vi "GetMethodExplicitName.vi"(8 "error in (no error)":errorcluster, 9 "options":i32 format="%.0x", 10 "method":string, 11 "Driver in":refnum<class "ViPER.lvclass">) -> (0 "error out":errorcluster, 1 "class explicit name":string, 2 "method explicit name":string, 3 "Driver out":refnum<class "ViPER.lvclass">, 4 "class":string, 5 "exists":bool, 6 "vi reference":refnum<vi>)   [LabVIEW 2022 SP3, in "ViPER.lvlib" / "ViPER.lvclass"]
doc: "### BSD License (http://www.opensource.org/licenses/bsd-license.php) Begin ###\n\nCopyright (c) 2018 Kurt Friday www.medulla.net\n\nAll rights reserved.\n\nRedistribution and use in source and binary forms, with or without\nmodification, are permitted provided that the following conditions are met:\n\n * Redistributions of source code must retain the above copyright\n notice, this list of conditions and the following disclaimer.\n\n * Redistributions in binary form must reproduce the above copyright\n notice, this list of conditions and the following disclaimer in the\n documentation and/or other materials provided with the distribution.\n\n * Neither the name of the <organization> nor the\n names of its contributors may be used to endorse or promote products\n derived from this software without specific prior written permission.\n\nTHIS SOFTWARE IS PROVIDED BY THE COPYRIGHT HOLDERS AND CONTRIBUTORS \"AS IS\" AND\nANY EXPRESS OR IMPLIED WARRANTIES, INCLUDING, BUT NOT LIMITED TO, THE IMPLIED\nWARRANTIES OF MERCHANTABILITY AND FITNESS FOR A PARTICULAR PURPOSE ARE\nDISCLAIMED. IN NO EVENT SHALL <COPYRIGHT HOLDER> BE LIABLE FOR ANY\nDIRECT, INDIRECT, INCIDENTAL, SPECIAL, EXEMPLARY, OR CONSEQUENTIAL DAMAGES\n(INCLUDING, BUT NOT LIMITED TO, PROCUREMENT OF SUBSTITUTE GOODS OR SERVICES;\nLOSS OF USE, DATA, OR PROFITS; OR BUSINESS INTERRUPTION) HOWEVER CAUSED AND\nON ANY THEORY OF LIABILITY, WHETHER IN CONTRACT, STRICT LIABILITY, OR TORT\n(INCLUDING NEGLIGENCE OR OTHERWISE) ARISING IN ANY WAY OUT OF THE USE OF THIS\nSOFTWARE, EVEN IF ADVISED OF THE POSSIBILITY OF SUCH DAMAGE."
uses:
  ViPER.lvclass
panel:
  # "### BSD License (http://www.opensource.org/licenses/bsd-license.php) Begin ###\n\nCopyright (c) 2018  Kurt Friday www.medulla.net\n\nAll rights reserved.\n\nRedistribution and use in source and binary forms, with or without\nmodification, are permitted provided that the following conditions are met:\n\n    * Redistributions of source code must retain the above copyright\n      notice, this list of conditions and the following disclaimer.\n\n    * Redistributions in binary form must reproduce the above copyright\n      notice, this list of conditions and the following disclaimer in the\n      documentation and/or other materials provided with the distribution.\n\n    * Neither the name of the <organization> nor the\n      names of its contributors may be used to endorse or promote products\n      derived from this software without specific prior written permission.\n\nTHIS SOFTWARE IS PROVIDED BY THE COPYRIGHT HOLDERS AND CONTRIBUTORS \"AS IS\" AND\nANY EXPRESS OR IMPLIED WARRANTIES, INCLUDING, BUT NOT LIMITED TO, THE IMPLIED\nWARRANTIES OF MERCHANTABILITY AND FITNESS FOR A PARTICULAR PURPOSE ARE\nDISCLAIMED. IN NO EVENT SHALL <COPYRIGHT HOLDER> BE LIABLE FOR ANY\nDIRECT, INDIRECT, INCIDENTAL, SPECIAL, EXEMPLARY, OR CONSEQUENTIAL DAMAGES\n(INCLUDING, BUT NOT LIMITED TO, PROCUREMENT OF SUBSTITUTE GOODS OR SERVICES;\nLOSS OF USE, DATA, OR PROFITS; OR BUSINESS INTERRUPTION) HOWEVER CAUSED AND\nON ANY THEORY OF LIABILITY, WHETHER IN CONTRACT, STRICT LIABILITY, OR TORT\n(INCLUDING NEGLIGENCE OR OTHERWISE) ARISING IN ANY WAY OUT OF THE USE OF THIS\nSOFTWARE, EVEN IF ADVISED OF THE POSSIBILITY OF SUCH DAMAGE."
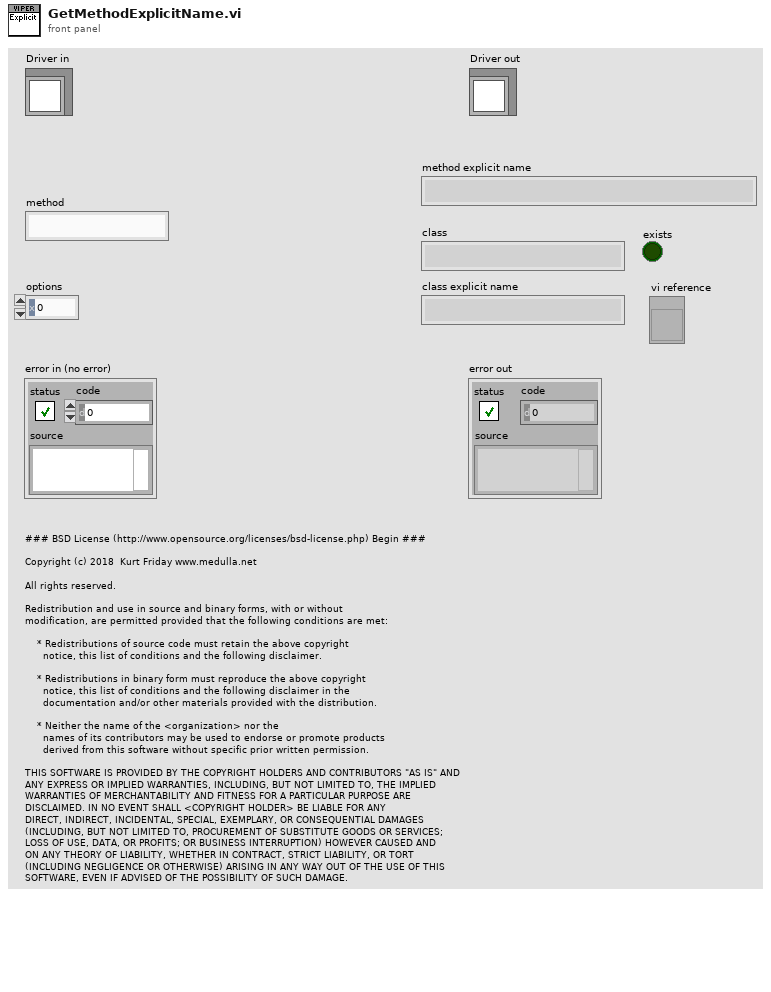
[diagram p1: front panel]
types:
  T1 = typedef "ViPER.lvlib/ViPER.lvclass/ObjectAttributes.ctl" = cluster{"Object":T2, "Ancestors":T4[], "Config":T5, "Init_OK":bool, "Hierachy":string[], "PPL?":bool[], "SFP_Open":bool[], "Config_SFP_Open":bool[], "SoftFP_event":refnum<user-event>[], "ConfigFP_event":refnum<user-event>[], "SoftFP_Shutdown_Notifier":refnum<notifier>[], "ConfigFP_Shutdown_Notifier":refnum<notifier>[]}
  T2 = typedef "ViPER.lvlib/ViPER.lvclass/ObjectDefinition.ctl" = cluster{"Name":string, "Ancestors":T3[]}
  T3 = typedef "ViPER.lvlib/ViPER.lvclass/Ancestor.ctl" = cluster{"Class":string, "Config":string, "Objects":string[]}
  T4 = typedef "ViPER.lvlib/ViPER.lvclass/ObjectLayers.ctl" = cluster{"Ancestor":string, "Objects":refnum<class "ViPER.lvclass">[], "Object_Names":string[], "Owned":bool[]}
  T5 = typedef "ViPER.lvlib/ViPER.lvclass/Config.ctl" = cluster{"default":string}
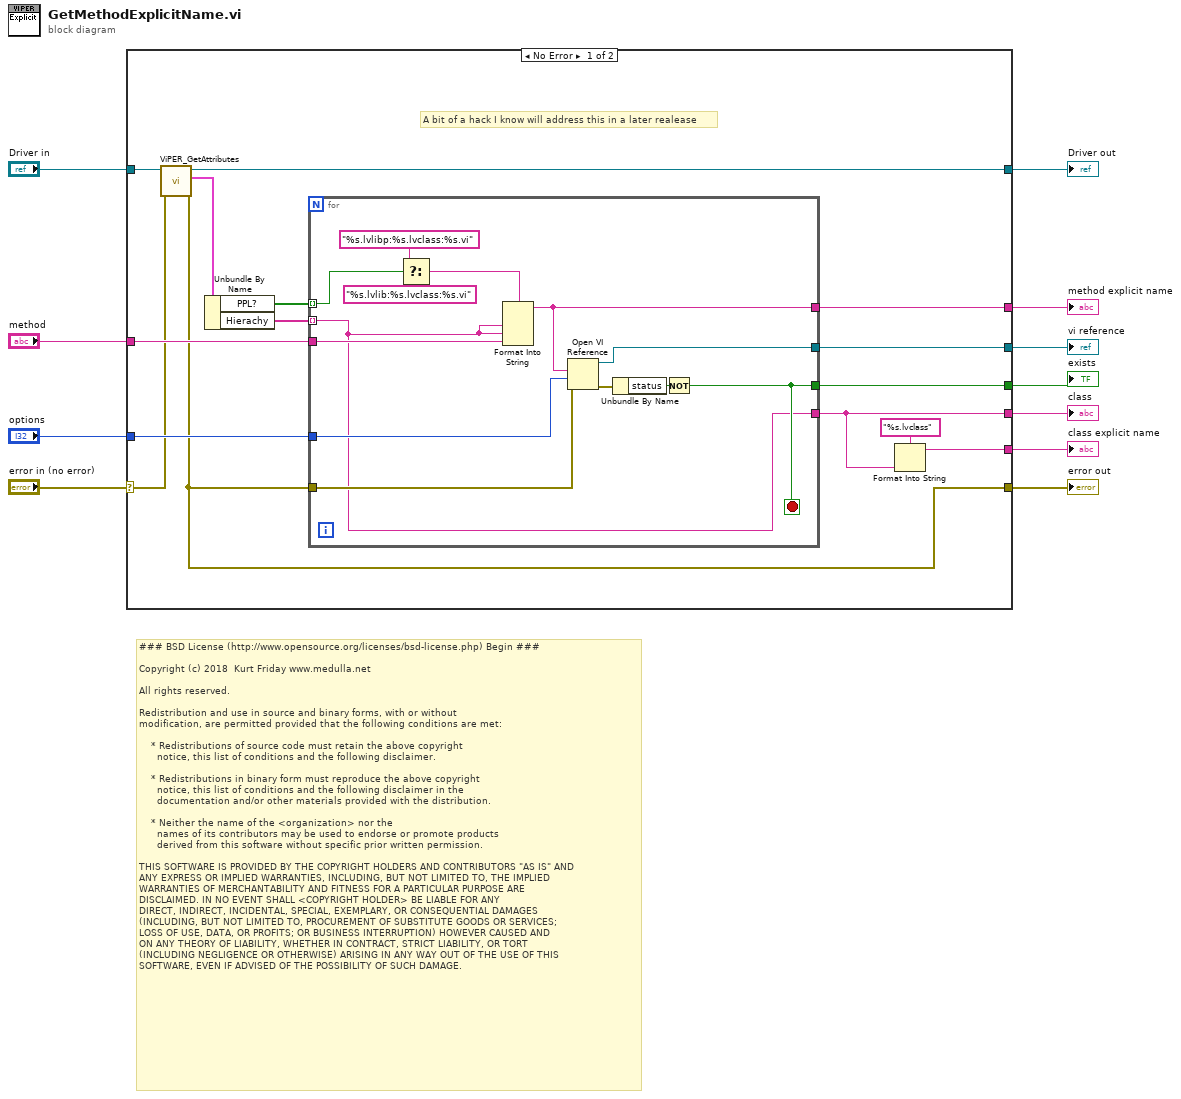
[diagram p0: block diagram]
diagram:
  # "### BSD License (http://www.opensource.org/licenses/bsd-license.php) Begin ###\n\nCopyright (c) 2018  Kurt Friday www.medulla.net\n\nAll rights reserved.\n\nRedistribution and use in source and binary forms, with or without\nmodification, are permitted provided that the following conditions are met:\n\n    * Redistributions of source code must retain the above copyright\n      notice, this list of conditions and the following disclaimer.\n\n    * Redistributions in binary form must reproduce the above copyright\n      notice, this list of conditions and the following disclaimer in the\n      documentation and/or other materials provided with the distribution.\n\n    * Neither the name of the <organization> nor the\n      names of its contributors may be used to endorse or promote products\n      derived from this software without specific prior written permission.\n\nTHIS SOFTWARE IS PROVIDED BY THE COPYRIGHT HOLDERS AND CONTRIBUTORS \"AS IS\" AND\nANY EXPRESS OR IMPLIED WARRANTIES, INCLUDING, BUT NOT LIMITED TO, THE IMPLIED\nWARRANTIES OF MERCHANTABILITY AND FITNESS FOR A PARTICULAR PURPOSE ARE\nDISCLAIMED. IN NO EVENT SHALL <COPYRIGHT HOLDER> BE LIABLE FOR ANY\nDIRECT, INDIRECT, INCIDENTAL, SPECIAL, EXEMPLARY, OR CONSEQUENTIAL DAMAGES\n(INCLUDING, BUT NOT LIMITED TO, PROCUREMENT OF SUBSTITUTE GOODS OR SERVICES;\nLOSS OF USE, DATA, OR PROFITS; OR BUSINESS INTERRUPTION) HOWEVER CAUSED AND\nON ANY THEORY OF LIABILITY, WHETHER IN CONTRACT, STRICT LIABILITY, OR TORT\n(INCLUDING NEGLIGENCE OR OTHERWISE) ARISING IN ANY WAY OUT OF THE USE OF THIS\nSOFTWARE, EVEN IF ADVISED OF THE POSSIBILITY OF SUCH DAMAGE."
  n1 = case shown="No Error" "error in (no error)" {
    selector: "error in (no error)" -> [w15 w41]
    tunnel: [w14 w41] -> w10
    tunnel: [w23 w40] -> w8
    tunnel: "Driver in" -> [w24 w40]
    tunnel: "method" -> [w21 _]
    tunnel: [w12 _] -> w6
    tunnel: [w16 _] -> w5
    tunnel: [w17 _] -> w4
    tunnel: [w26 _] -> w3
    tunnel: "options" -> [w25 _]
    tunnel: [w19 _] -> w1
    frame No Error {
      # "A bit of a hack I know will address this in a later realease"
      n2 = call "ViPER_GetAttributes.vi"("error in (no error)"=w15, "reference in"=w24) -> ("error out"=w14:errorcluster, "Data"=w22:T1, "reference out"=w23:refnum<class "ViPER.lvclass">)  [unwired: 6 in, 1 out]
      n3 = Unbundle By Name(w22) -> ("PPL?"=w13:bool[], "Hierachy"=w18:string[])
      n4 = for {
        tunnel: [w34] -> w16
        tunnel: [w39] -> w26
        tunnel: w25 -> [w38]
        tunnel: [w35] -> w17
        tunnel: w18 -> [w34] mode=indexing
        tunnel: w21 -> [w37]
        tunnel: w14 -> [w36]
        tunnel: [w27] -> w12
        tunnel: w13 -> [w33] mode=indexing
        stop <- w35 stop-if-true
        n5 = Select(t="%s.lvlibp:%s.lvclass:%s.vi", s=w33, f="%s.lvlib:%s.lvclass:%s.vi") -> (s? t:f=w28:string)
        n6 = Format Into String(format string=w28, w34, w34, w37) -> (resulting string=w27:string)  [unwired: 2 in, 1 out]
        n7 = Open VI Reference(vi path=w27, options=w38, error in (no error)=w36) -> (vi reference=w39:refnum<vi>, error out=w32:errorcluster)  [unwired: 3 in]
        n8 = Unbundle By Name(w32) -> ("status"=w31:bool)
        n9 = Not(x=w31) -> (.not. x?=w35:bool)
      }
      n10 = Format Into String(format string="%s.lvclass" ("regular expression"), w16) -> (resulting string=w19:string)  [unwired: 2 in, 1 out]
    }
    frame Error {
    }
  }
  "error out" <- w10
  "Driver out" <- w8
  "method explicit name" <- w6
  "class" <- w5
  "class explicit name" <- w1
  "exists" <- w4
  "vi reference" <- w3
